vi "_086.vi"() -> ()   [LabVIEW 2024]
panel:
  out "output array":i32[][](array[numeric])
  out "size(s)":i32
  in  "array":dbl[](array[numeric])
  out "initialized array":i32[](array[numeric])
  out "Array 2":i32[](array[numeric])
  out "Array":i32[](array[numeric])
  # "Fundamentals :"
  # "15~>After running this VI,what is the value displayed in the o/p ?"
  # "Nrml Approach :"
  # "Dfrnt Approach :"
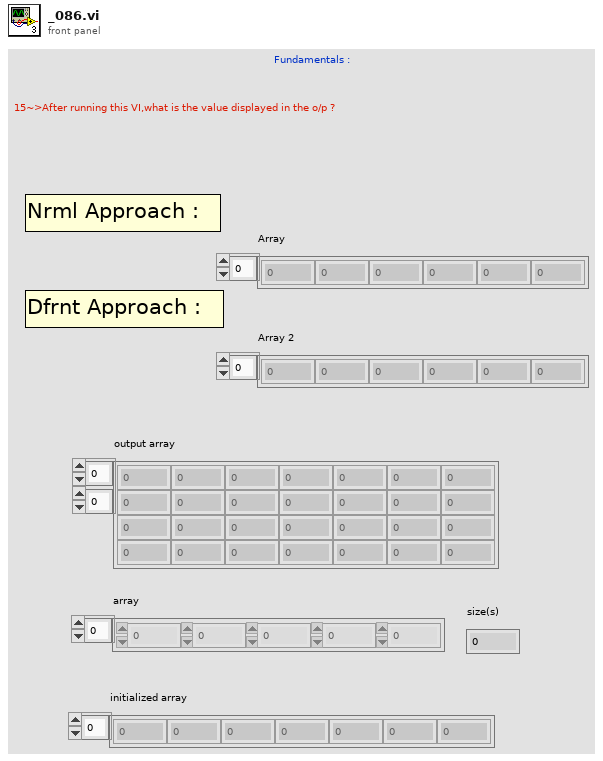
[diagram p1: front panel]
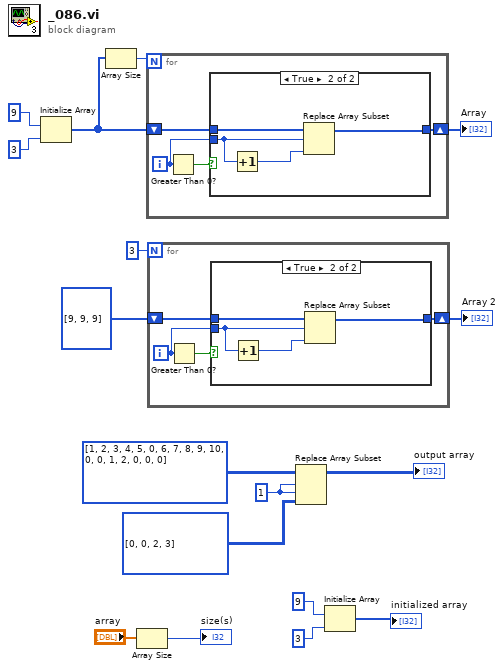
[diagram p0: block diagram]
diagram:
  w1 = 1
  n1 = Initialize Array "Initialize Array"(9, 3) -> (w16:i32[])
  n2 = Array Size(array=w16) -> (size(s)=w15:i32)
  n3 = Array Size(array="array") -> (size(s)=→"size(s)":i32)
  n4 = for {
    N: w15 -> [_]
    shift-right: [w20] -> w14
    shift-left: w16 -> [w21]
    i -> [w18]
    n5 = Greater Than 0?(x=w18) -> (x > 0?=w19:bool)
    n6 = case shown="True" w19 {
      tunnel: w21 -> [w22 w26]
      tunnel: [w22 w25] -> w20
      tunnel: w18 -> [_ w24]
      frame False {
      }
      frame True {
        n7 = Increment(x=w24) -> (x+1=w23:i32)
        n8 = Replace Array Subset "Replace Array Subset"(array=w26, new element=w23, index=w24) -> (w25:i32[])
      }
    }
  }
  "Array" <- w14
  n9 = for {
    N: 3 -> [_]
    shift-right: [w29] -> w12
    shift-left: i32[] [9, 9, 9] -> [w30]
    i -> [w27]
    n10 = Greater Than 0?(x=w27) -> (x > 0?=w28:bool)
    n11 = case shown="True" w28 {
      tunnel: w30 -> [w31 w35]
      tunnel: [w31 w34] -> w29
      tunnel: w27 -> [_ w33]
      frame False {
      }
      frame True {
        n12 = Increment(x=w33) -> (x+1=w32:i32)
        n13 = Replace Array Subset "Replace Array Subset"(array=w35, new element=w32, index=w33) -> (w34:i32[])
      }
    }
  }
  "Array 2" <- w12
  n14 = Replace Array Subset "Replace Array Subset"(array=i32[][] [[1, 2, 3, 4, 5, 0], [6, 7, 8, 9, 10, 0], [0, 1, 2, 0, 0, 0]], new element=i32[][] [[0, 0], [2, 3]], index (row)=w1, index (col)=w1) -> (→"output array":i32[][])
  n15 = Initialize Array "Initialize Array"(9, 3) -> (→"initialized array":i32[])
